vi "Re-Init Test State.vi"(0 ".NET Refnum in":refnum<k24>, 11 "error in (no error)":errorcluster) -> (15 "error out":errorcluster)   [LabVIEW 2016]
doc: "This VI"
uses:
  C:/Automation/DLLs/PC Dot Net/GeaCommunication.dll
  Common/LabVIEW GEA2 Toolkit/LabVIEW_GEA2_Toolkit.lvlibp/type defs/ERD Write Data In.ctl
  Common/LabVIEW GEA2 Toolkit/LabVIEW_GEA2_Toolkit.lvlibp/type defs/Data Type.ctl
  Common/LabVIEW GEA2 Toolkit/LabVIEW_GEA2_Toolkit.lvlibp/type defs/Source_Destination.ctl
  Common/LabVIEW GEA2 Toolkit/LabVIEW_GEA2_Toolkit.lvlibp
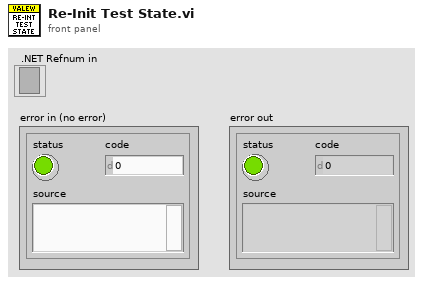
[diagram p1: front panel]
types:
  T1 = typedef "LabVIEW_GEA2_Toolkit.lvlibp/Source_Destination.ctl" = cluster{"Source":u8, "Destination":u8}
  T2 = typedef "LabVIEW_GEA2_Toolkit.lvlibp/ERD Write Data In.ctl" = cluster{"ERD Number":u16, "Data Type":T3, "Data":string}
  T3 = typedef "LabVIEW_GEA2_Toolkit.lvlibp/Data Type.ctl" = enum16{"string", "boolean", "uint8_t", "uint16_t", "uint32_t", "uint64_t", "int8_t", "int16_t", "int32_t", "int64_t"}
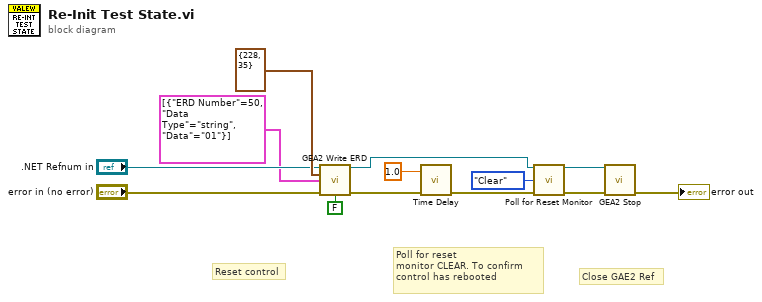
[diagram p0: block diagram]
diagram:
  # "Close GAE2 Ref"
  # "Reset control"
  # "Poll for reset\nmonitor CLEAR. To confirm\ncontrol has rebooted"
  n1 = call "GEA2 Write ERD.vi"("GEA2 Reference In"=".NET Refnum in", "GEA Inputs"=T1 {"Source"=228, "Destination"=35}, "Write ERD List"=T2[] [{"ERD Number"=50, "Data Type"=enum."string", "Data"="01"}], "Error In"="error in (no error)", "Verify ERD Response?"=FALSE) -> ("GEA2 Reference Out"=w2:refnum<k24>, "Error Out"=w7:errorcluster)  [unwired: 8 in, 1 out]
  n2 = call "Time Delay"("error in (no error)"=w7, "Delay Time (s)"=1.0) -> ("error out"=w4:errorcluster)  [unwired: 9 in]
  n3 = call "Poll for Reset Monitor.vi"("GEA2 Reference In"=w2, "Status"=enum16{"Clear", "Set"}."Clear", "Error In"=w4) -> ("GEA2 Reference Out"=w1:refnum<k24>, "Error Out"=w3:errorcluster)  [unwired: 8 in, 3 out]
  n4 = call "GEA2 Stop.vi"("GEA2 Reference In"=w1, "Error In"=w3) -> ("Error Out"=→"error out":errorcluster)  [unwired: 13 in]
